vi "HandleObservationSync.vi"(8 "error in (no error)":errorcluster, 11 "S4GUI in":refnum<class "S4GUI.lvclass">) -> (0 "error out":errorcluster, 3 "S4GUI out":refnum<class "S4GUI.lvclass">)   [LabVIEW 2018, in "S4GUI.lvclass"] (continued)
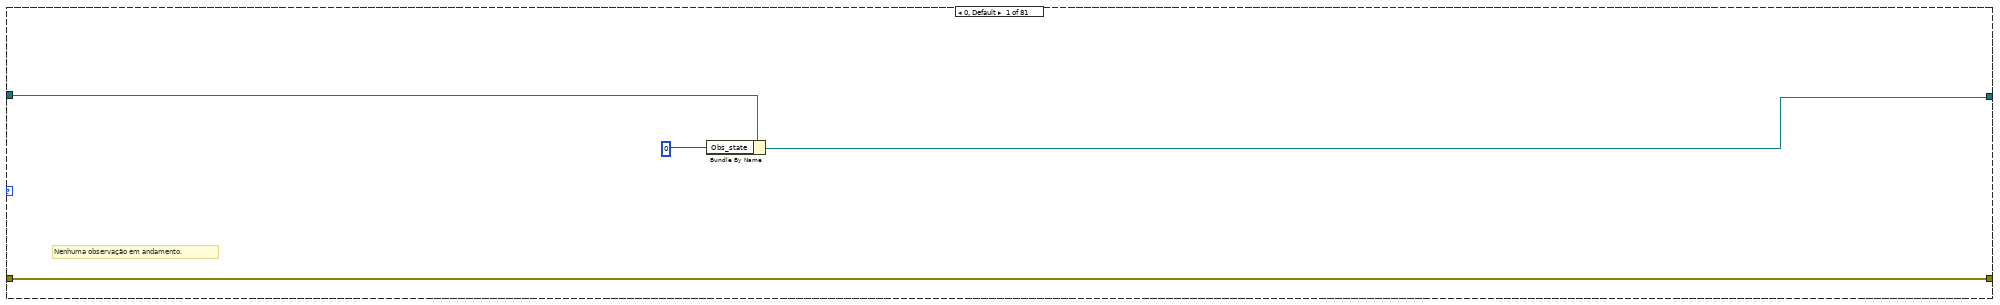
[diagram p2: hidden frame]
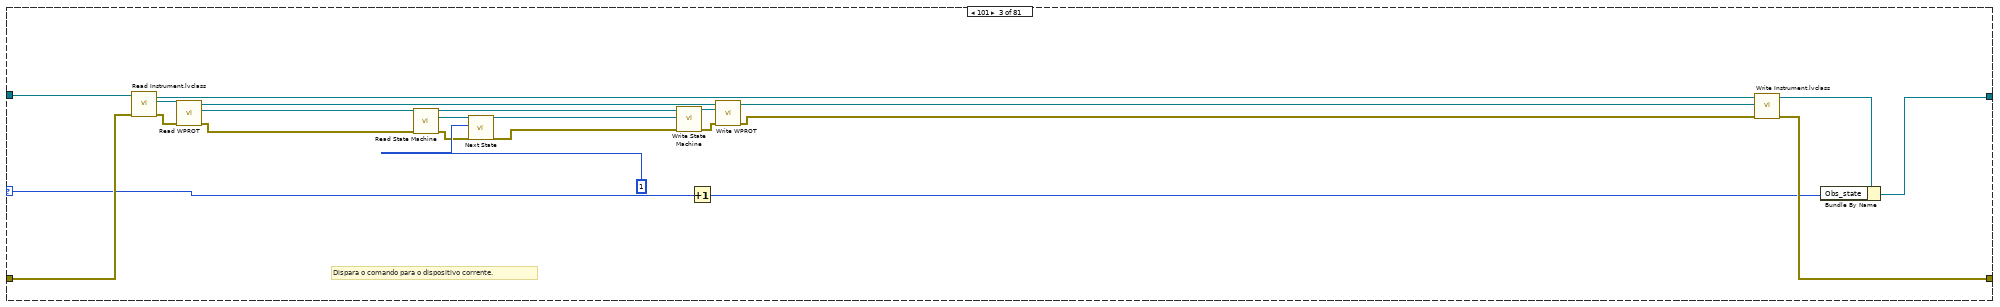
[diagram p4: hidden frame]
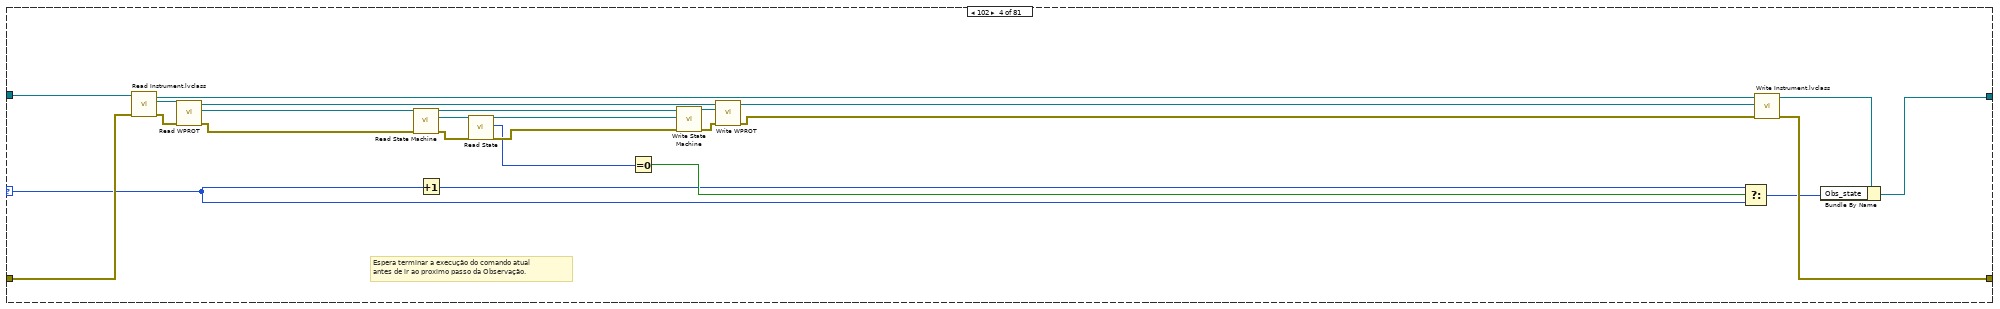
[diagram p5: hidden frame]
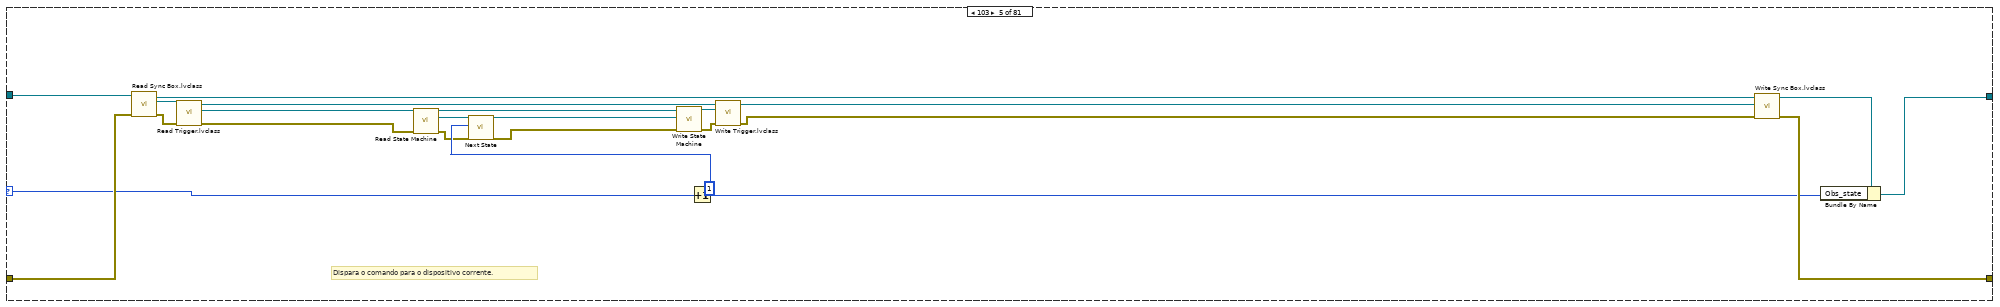
[diagram p6: hidden frame]
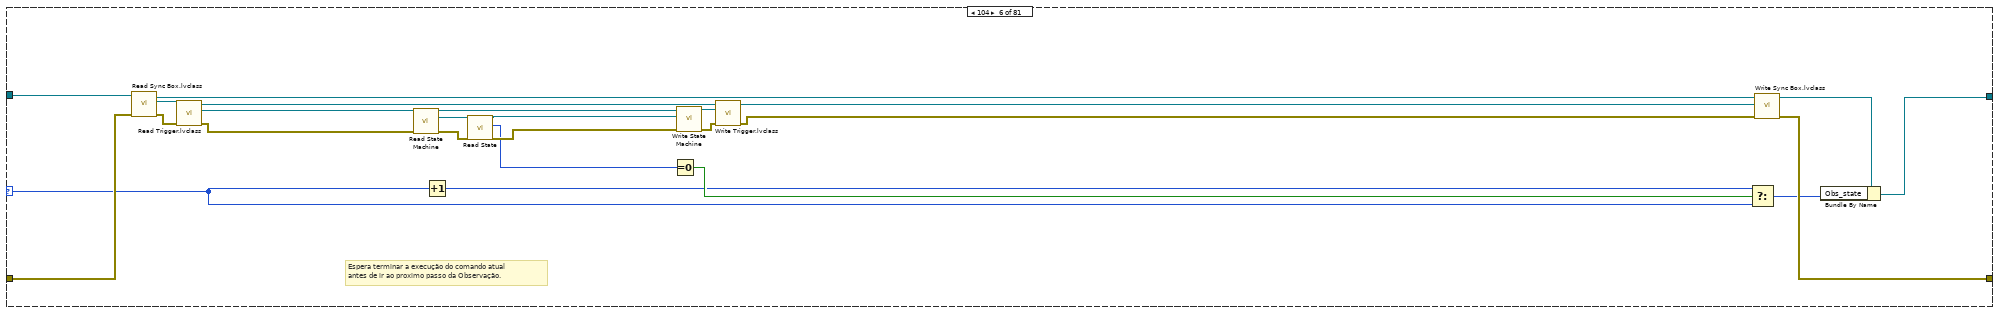
[diagram p7: hidden frame]
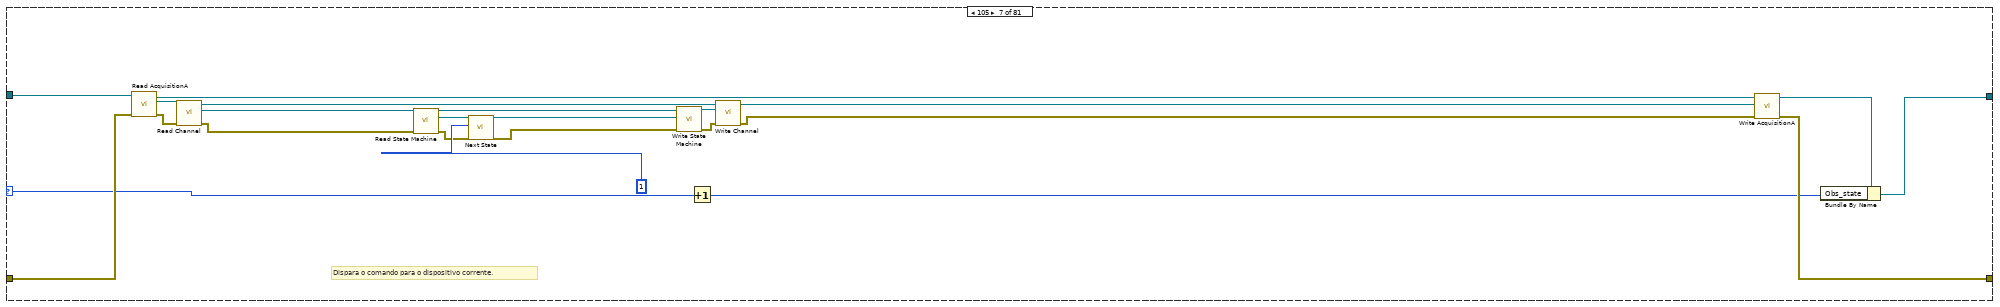
[diagram p8: hidden frame]
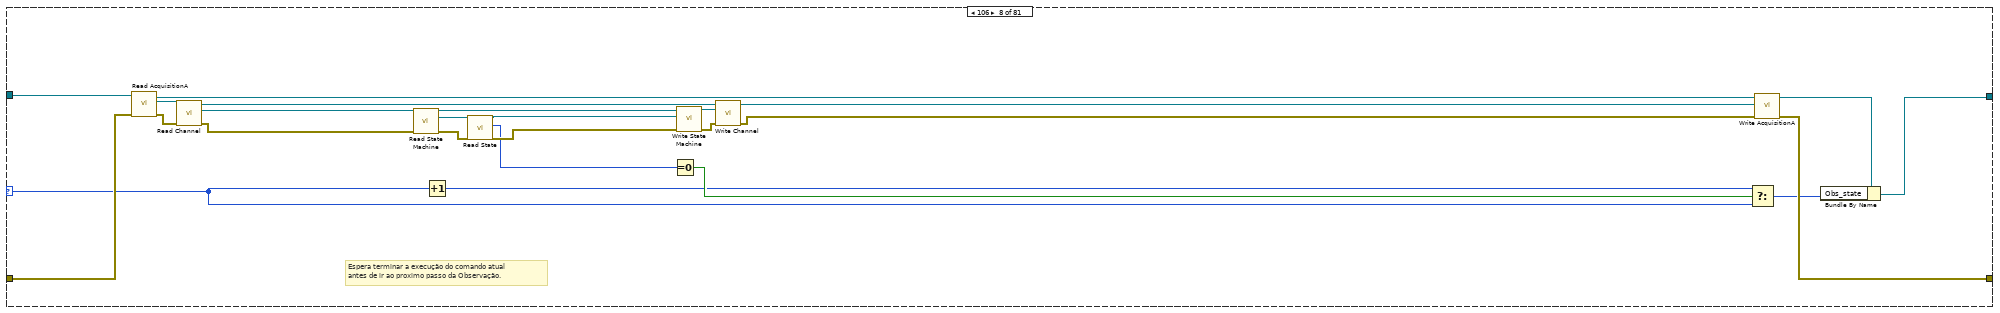
[diagram p9: hidden frame]
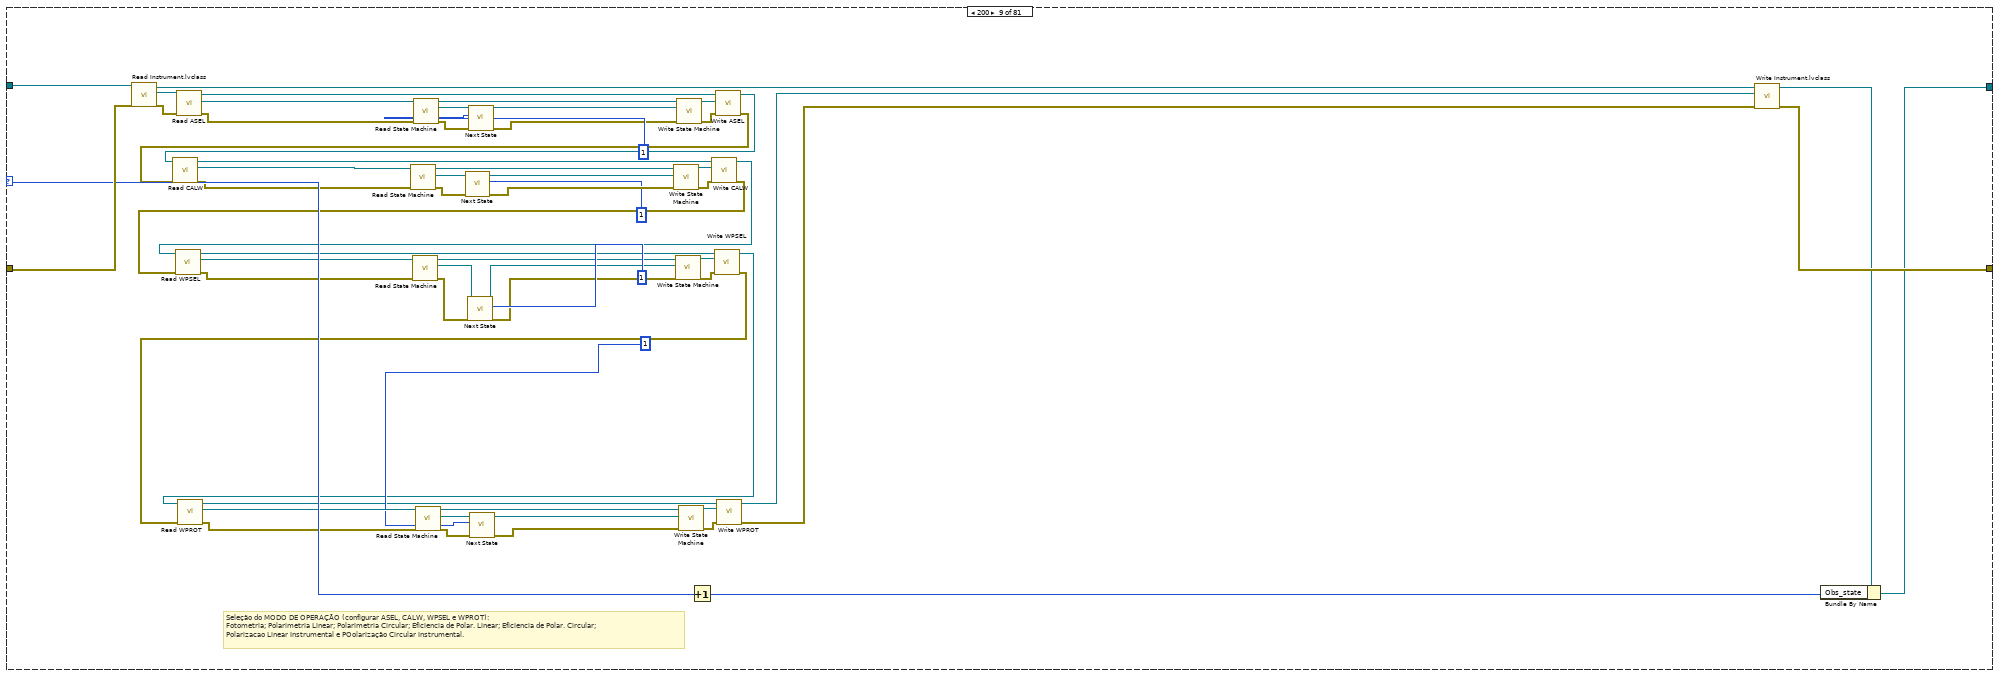
[diagram p10: hidden frame]
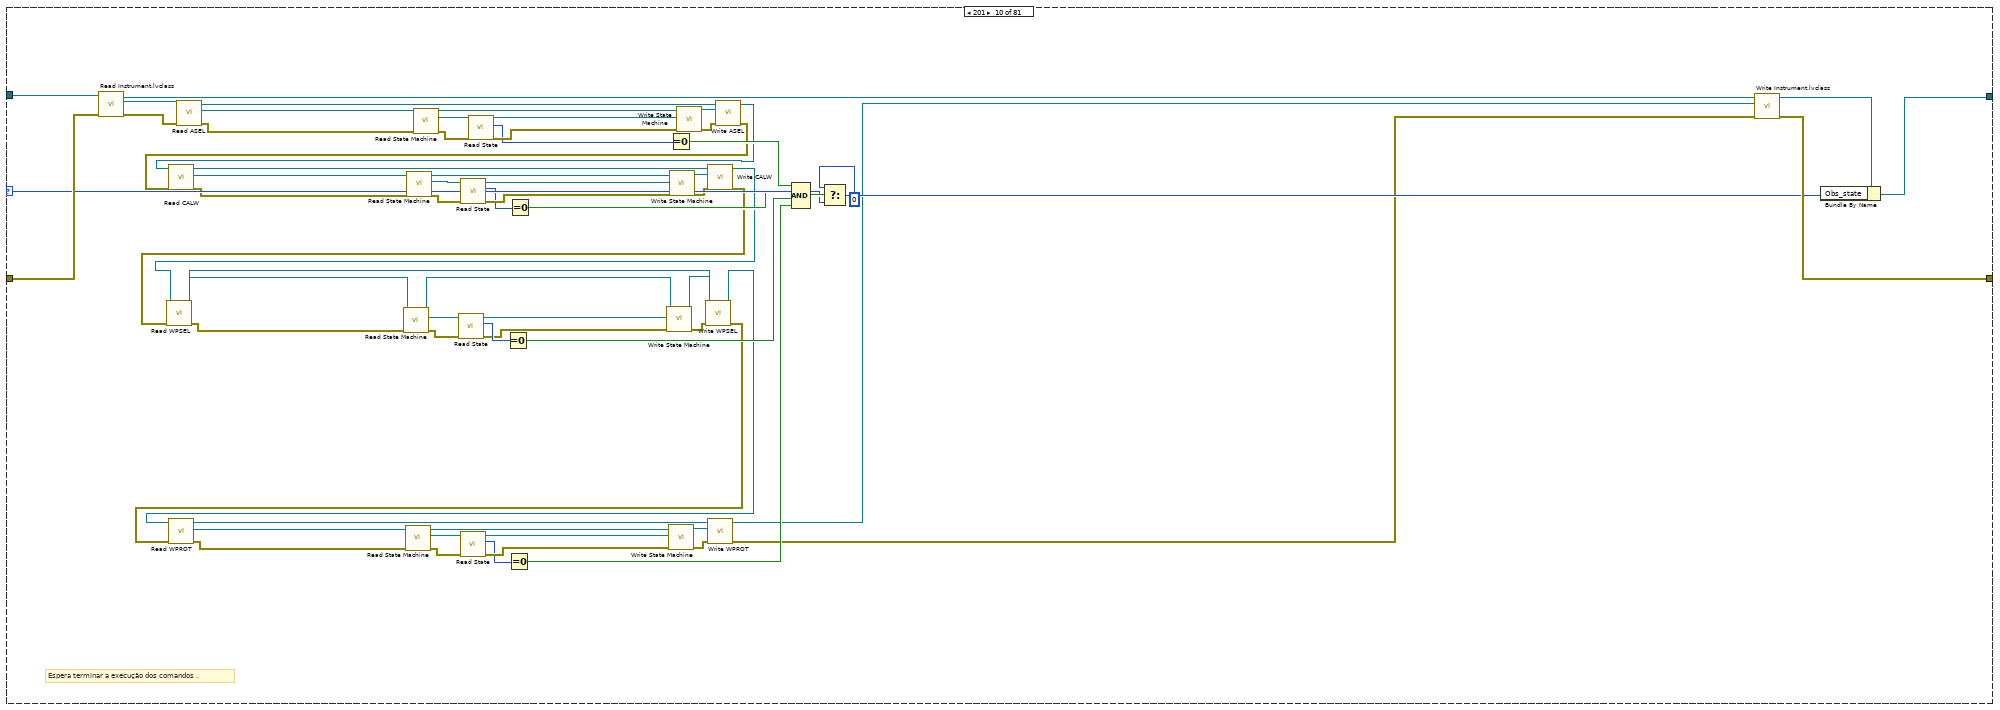
[diagram p11: hidden frame]
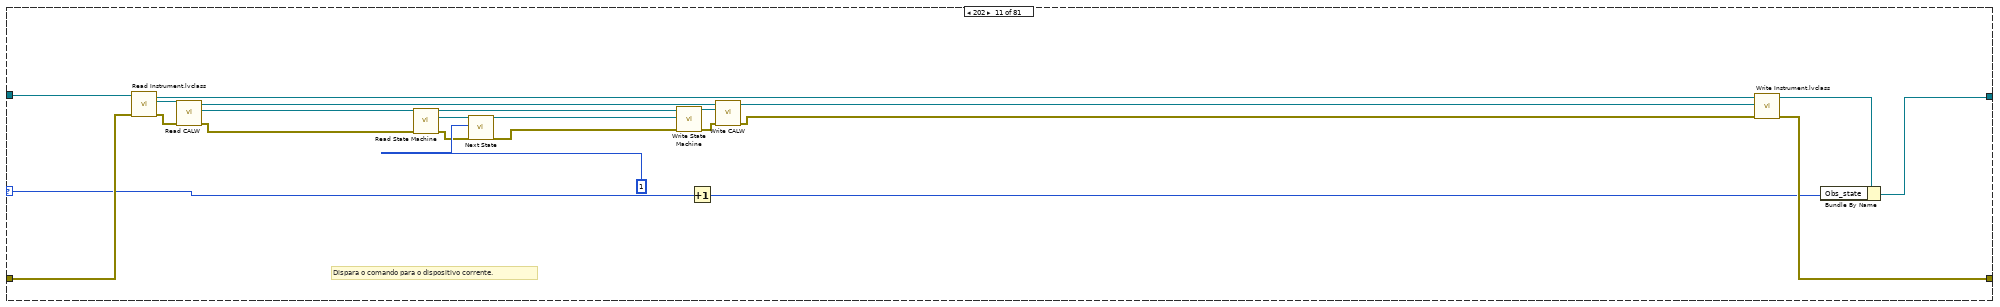
[diagram p12: hidden frame]
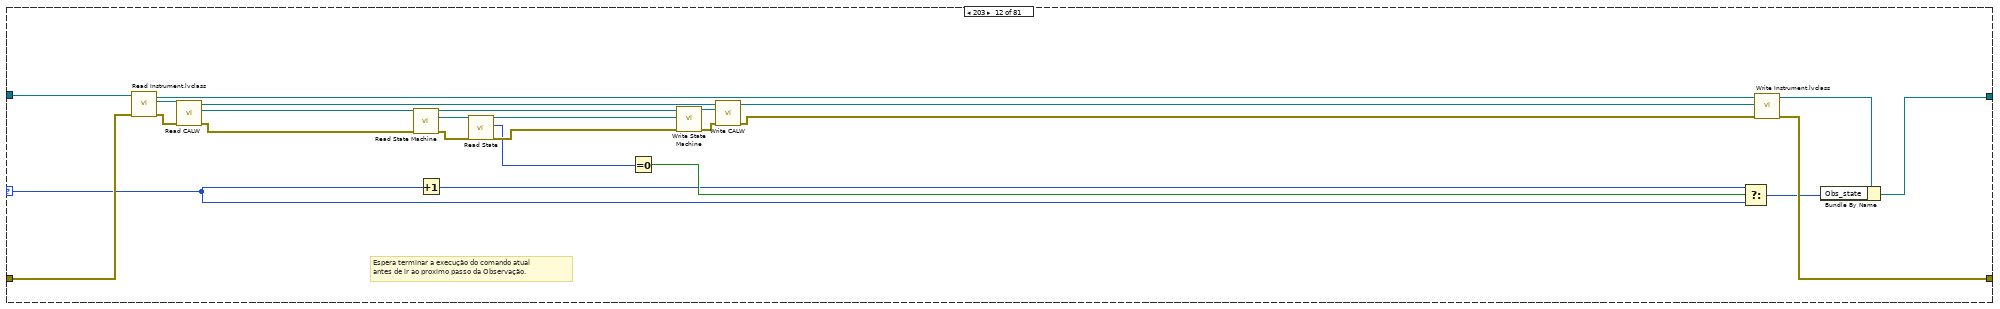
[diagram p13: hidden frame]
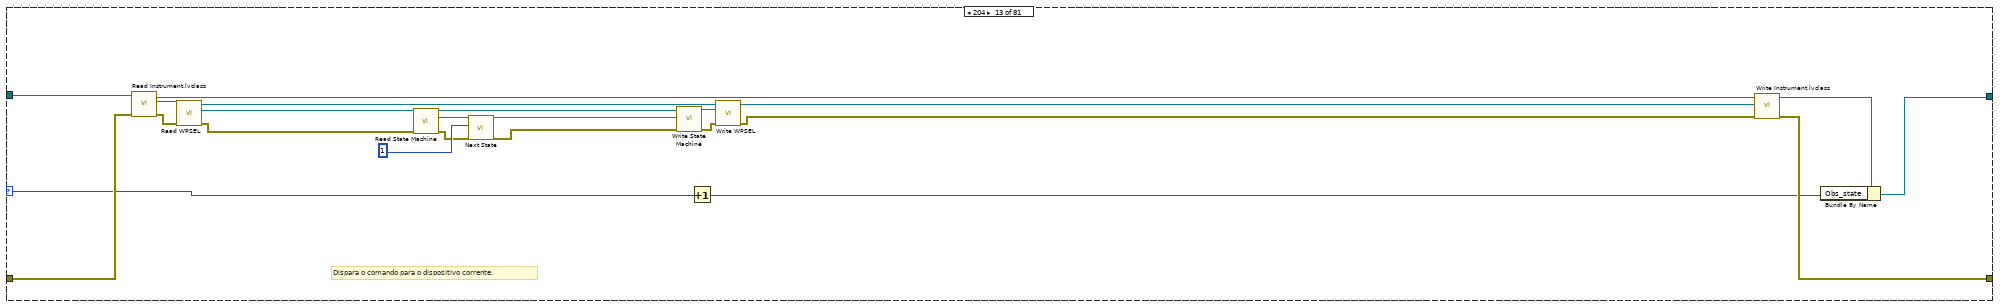
[diagram p14: hidden frame]
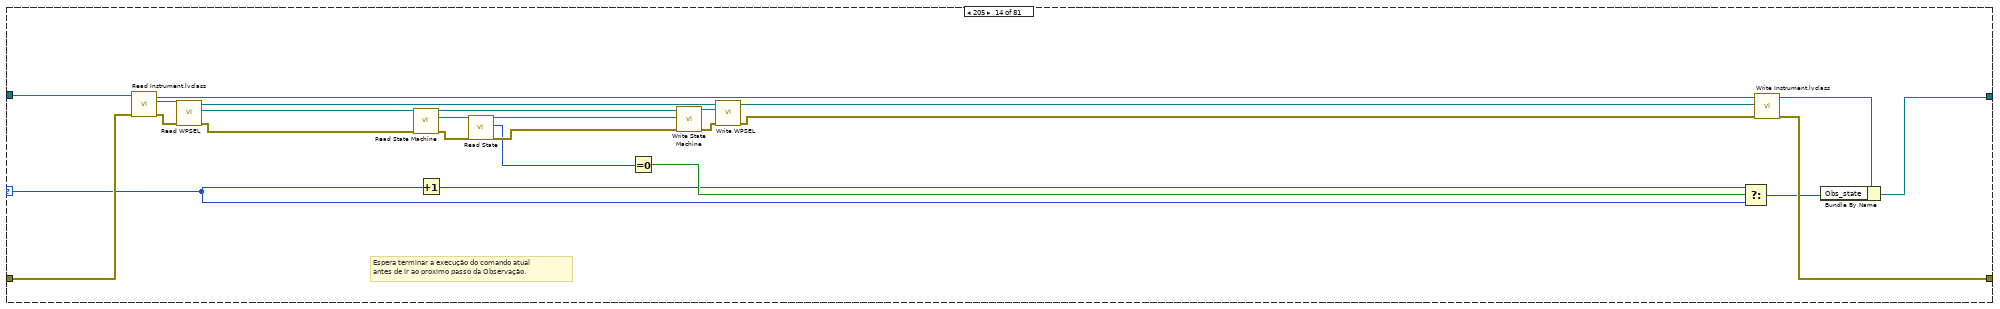
[diagram p15: hidden frame]
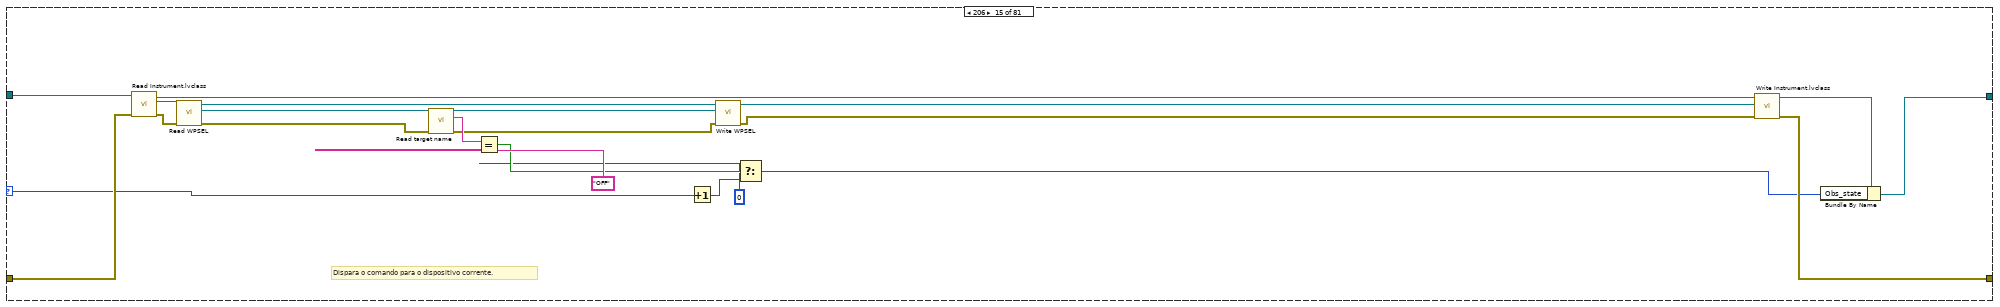
[diagram p16: hidden frame]
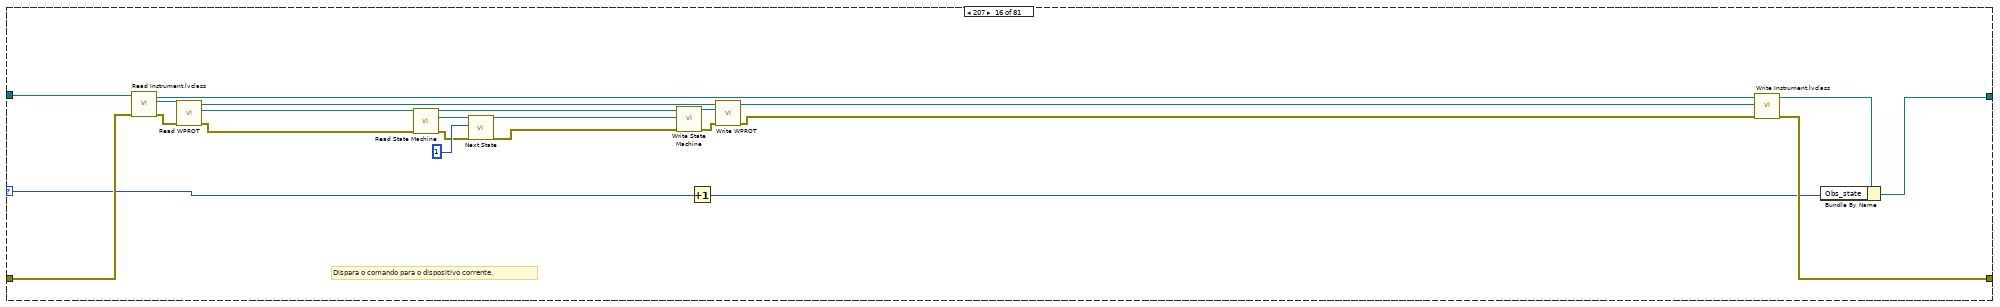
[diagram p17: hidden frame]
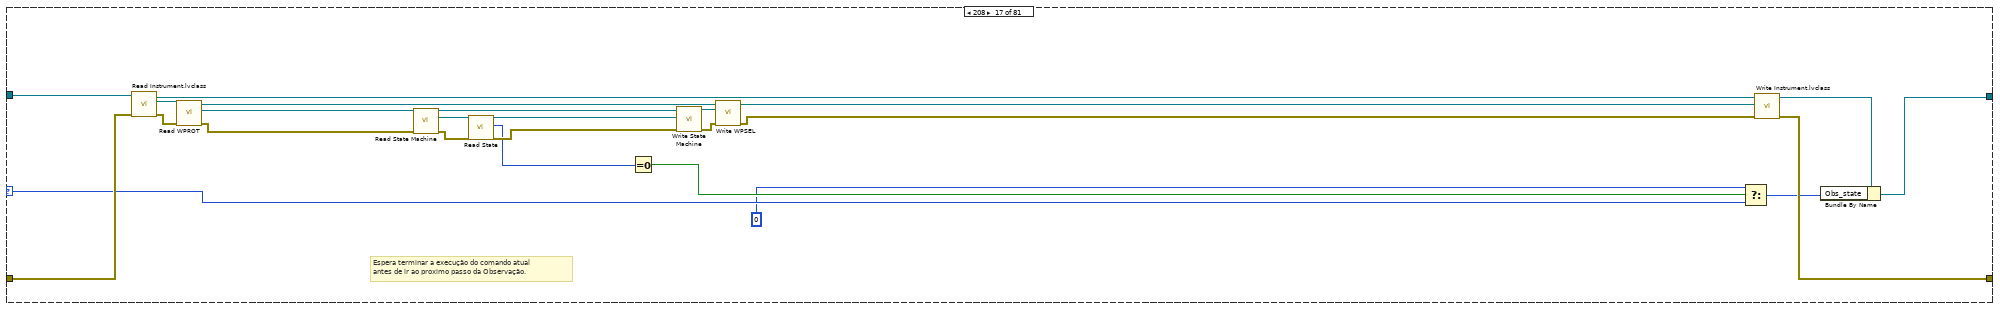
[diagram p18: hidden frame]
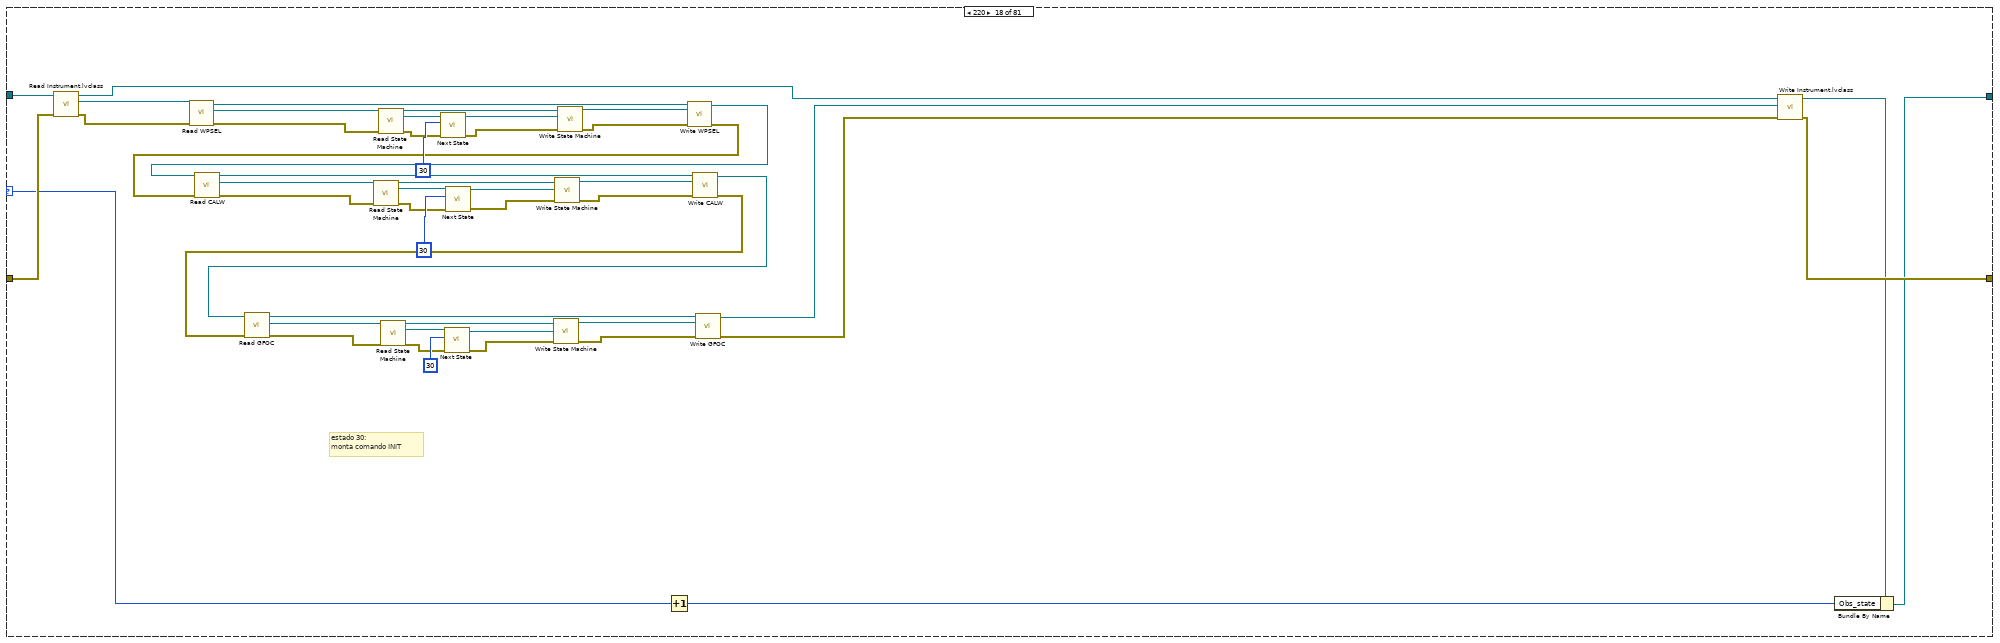
[diagram p19: hidden frame]
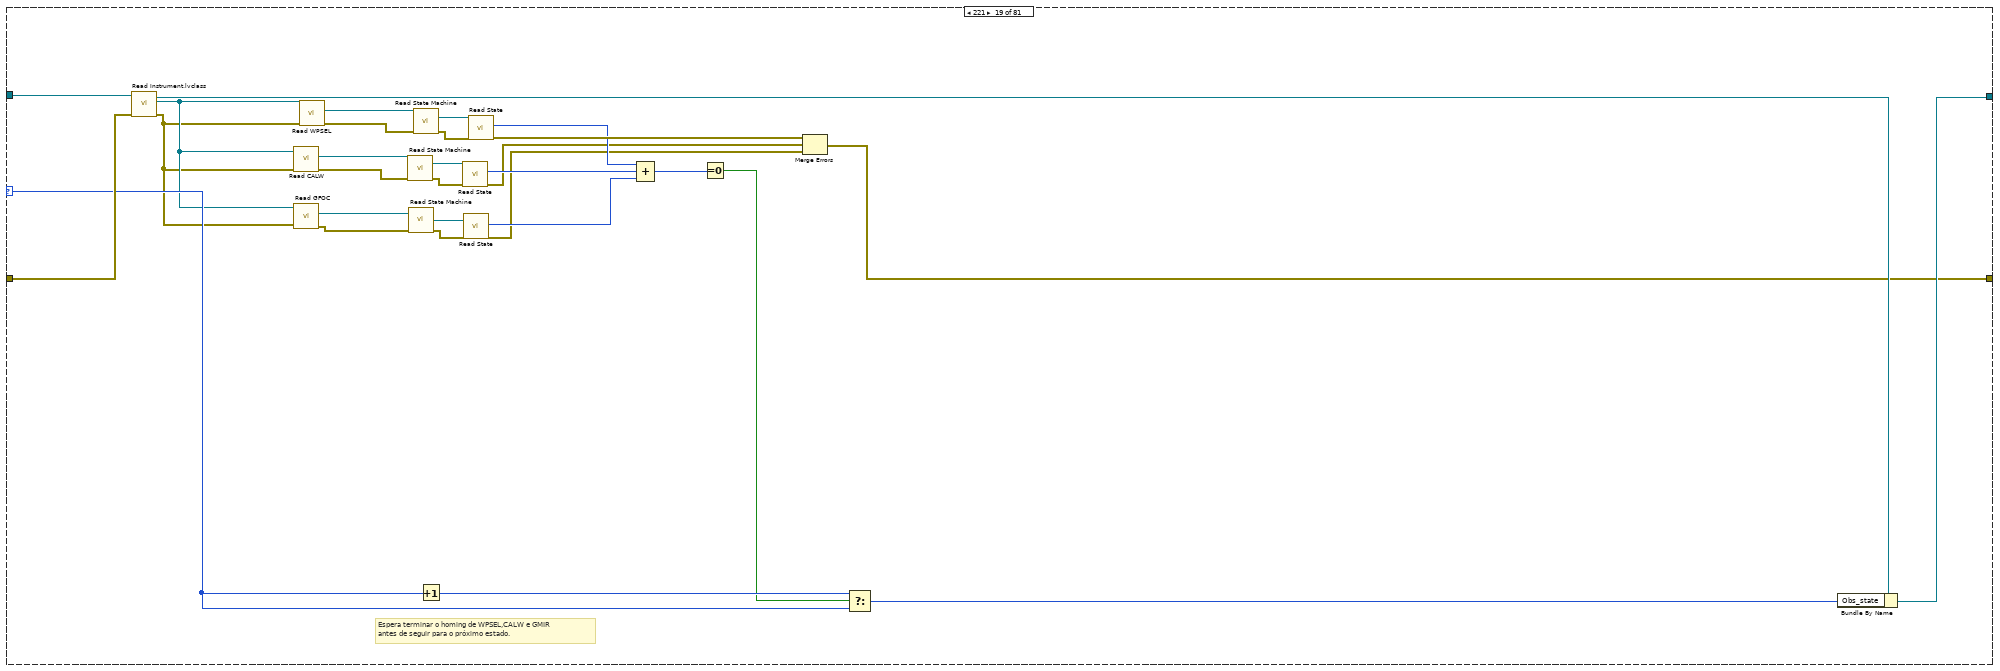
[diagram p20: hidden frame]
                      n2099 = Bundle By Name(cluster=w5793, "Obs_state"=w5790, "sequesDone"=w5789, "cyclesDone"=w5789) -> (w5792:refnum<class "S4GUI.lvclass">)
                    }
                  }
                }
              }
            }
          }
        }
        frame 368 {
          n2100 = Unbundle By Name(w5895) -> ("TelFocus.lvclass"=w5894:refnum<class "TelFocus.lvclass">)
          n2101 = call-dynamic "VerifSteps.vi"("error in (no error)"=w5891, "TelFocus in"=w5894) -> ("error out"=w5890:errorcluster, "continua?"=w5896:bool, "TelFocus out"=w5893:refnum<class "TelFocus.lvclass">)  [unwired: 7 in]
          n2102 = Bundle By Name(cluster=w5895, "TelFocus.lvclass"=w5893) -> (w5892:refnum<class "S4GUI.lvclass">)
          n2103 = Select(t=u32 360, s=w5896, f=u32 0) -> (s? t:f=w5899:u32)
          n2104 = Bundle By Name(cluster=w5892, "Obs_state"=w5899) -> (w5900:refnum<class "S4GUI.lvclass">)
        }
        frame 400 {
          # "Estado de \"Pause\": fica parado aqui até o botão START seja pressionado."
        }
        frame 500 {
          # "Espera terminar o envio de RESUME para todos os ACS."
          # "Estado de \"Pause\": fica parado aqui até o botão START seja pressionado."
          n2105 = call-dynamic "VerifyAcqIdle.vi"("error in (no error)"=w5905, "S4GUI in"=w5909) -> ("error out"=w5904:errorcluster, "idle"=w5908:bool, "S4GUI out"=w5907:refnum<class "S4GUI.lvclass">)  [unwired: 6 in, 1 out]
          n2106 = case shown="True" w5908 {
            tunnel: w5907 -> [w5911 w5921]
            tunnel: [w5911 w5913] -> w5906
            tunnel: w5904 -> [w5910 w5920]
            tunnel: [w5910 w5914] -> w5903
            frame False {
            }
            frame True {
              n2107 = call-dynamic "LoadPrevAcqRunState.vi"("error in (no error)"=w5920, "S4GUI in"=w5921) -> ("error out"=w5915:errorcluster, "S4GUI out"=w5916:refnum<class "S4GUI.lvclass">)  [unwired: 8 in]
              n2108 = Tick Count (ms)() -> (millisecond timer value=w5912:u32)
              n2109 = call-dynamic "Read Obs_prevstate.vi"("error in (no error)"=w5915, "S4ACS_GUI in"=w5916) -> ("error out"=w5919:errorcluster, "Obs_prevstate"=w5917:u32, "S4ACS_GUI out"=w5918:refnum<class "S4GUI.lvclass">)  [unwired: 7 in]
              n2110 = local write "time307"(w5912) -> ()
              n2111 = local write "time1"(w5912) -> ()
              n2112 = call-dynamic "Write Obs_state.vi"("error in (no error)"=w5919, "Obs_state"=w5917, "S4ACS_GUI in"=w5918) -> ("error out"=w5914:errorcluster, "S4ACS_GUI out"=w5913:refnum<class "S4GUI.lvclass">)  [unwired: 7 in]
            }
          }
        }
      }
    }
    frame Error {
    }
  }
  "error out" <- w3
  "S4GUI out" <- w2
